vi "svx_Orbit Exec Commands.vi"(4 "Display State In":T2={"X Scale"={"Name"="Horizontal", "FString"="%#.2g", "Major Color"=16777238, "Minor Color"=16777216, "Scale Visible"=TRUE, " Label Visible"=TRUE, "Grid Style"=1}, "Y Scale"={"Name"="Vertical", "FString"="%#.2g", "Major Color"=16777238, "Minor Color"=16777216, "Scale Visible"=TRUE, " Label Visible"=TRUE, "Grid Style"=1}, "Plot"={"Point Style"=0, "Line Width"=0, "Line Style"=0, "Plot Color"=9727, "Point/fill"=0}, "Arrow/Crosshair Color"=9727, "Tacho Point Color"=16711680, "Container Bounds"={"Width"=563, "Height"=294}, "Axis Maximum"=10.0, "Probe Angles"={"Angle X"=0.0, "Angle Y"=1.5707963267948966}, "Background Color"=16777226, "Cursor"={"Cursor Point Style"=13, "Cursor Style"=4, "Cursor Line Width"=1, "Cursor Line Style"=0, "Cursor Color"=9727, "Cursor Name Visible"=TRUE, "Cursor Visible"=TRUE, "Cursor Position"={"X"=0.0, "Y"=0.0}, "Cursor Index"=0, "Cursor Lock"=FALSE}, "Elliptical Info"=[], "Legend Visible"=TRUE, "Scale Range Change"=refnum, "Strings[]"={"Custom pair name"=FALSE, "Row Strings []"=[], "Column Strings []"=[]}, "Index"=[{"pair index"=0, "order index"=0}], " Parents Tags"=[], "Children Tags"=[], "Open?"=[], "Label"="", "Legend Width"=120, "Pair Strings Changed?"=FALSE, "Size"=[], "Legend Background"=16777226, "Legend Font"=16777222, "Cursor Release"=refnum, "Autoscale"=TRUE, "Precession Direction"=[], "Item Width"=0, "User Pair Strings []"=[], "Users Order Strings []"=[], "Autoscale Once"=TRUE, "Property Write"=refnum} caption="State" {"Index"."order index" min=0; "Index"."pair index" min=0; "Axis Maximum" min=0.0}, 5 "Data In":T4, 6 "Commands":T1[](array[typedef]), 7 "Container":refnum<vi>, 8 "Facade VI":refnum<vi>, 9 "Cursor Info":refnum<vi>, 10 "Tree":refnum<vi>, 11 "Orbit Plot":refnum<vi>) -> (0 "Display State Out":T2={"X Scale"={"Name"="Horizontal", "FString"="%#.2g", "Major Color"=16777238, "Minor Color"=16777216, "Scale Visible"=TRUE, " Label Visible"=TRUE, "Grid Style"=1}, "Y Scale"={"Name"="Vertical", "FString"="%#.2g", "Major Color"=16777238, "Minor Color"=16777216, "Scale Visible"=TRUE, " Label Visible"=TRUE, "Grid Style"=1}, "Plot"={"Point Style"=0, "Line Width"=0, "Line Style"=0, "Plot Color"=9727, "Point/fill"=0}, "Arrow/Crosshair Color"=9727, "Tacho Point Color"=16711680, "Container Bounds"={"Width"=563, "Height"=294}, "Axis Maximum"=10.0, "Probe Angles"={"Angle X"=0.0, "Angle Y"=1.5707963267948966}, "Background Color"=16777226, "Cursor"={"Cursor Point Style"=13, "Cursor Style"=4, "Cursor Line Width"=1, "Cursor Line Style"=0, "Cursor Color"=9727, "Cursor Name Visible"=TRUE, "Cursor Visible"=TRUE, "Cursor Position"={"X"=0.0, "Y"=0.0}, "Cursor Index"=0, "Cursor Lock"=FALSE}, "Elliptical Info"=[], "Legend Visible"=TRUE, "Scale Range Change"=refnum, "Strings[]"={"Custom pair name"=FALSE, "Row Strings []"=[], "Column Strings []"=[]}, "Index"=[{"pair index"=0, "order index"=0}], " Parents Tags"=[], "Children Tags"=[], "Open?"=[], "Label"="", "Legend Width"=120, "Pair Strings Changed?"=FALSE, "Size"=[], "Legend Background"=16777226, "Legend Font"=16777222, "Cursor Release"=refnum, "Autoscale"=TRUE, "Precession Direction"=[], "Item Width"=0, "User Pair Strings []"=[], "Users Order Strings []"=[], "Autoscale Once"=TRUE, "Property Write"=refnum} caption="State" {"Index"."order index" min=0; "Index"."pair index" min=0; "Axis Maximum" min=0.0})   [LabVIEW 2017, in "SVX Orbit.xctl"]
uses:
  <vilib>/addons/_XControls/Orbit Plot/SVX Orbit.xctl
  <vilib>/addons/_XControls/Orbit Plot/subVIs/svx_Orbit Data.ctl
  <vilib>/addons/_XControls/Orbit Plot/subVIs/svx_Orbit Internal State.ctl
  <vilib>/addons/_XControls/Orbit Plot/subVIs/svx_Orbit Bounds.ctl
  <vilib>/addons/_XControls/Orbit Plot/subVIs/svx_Orbit Core States.ctl
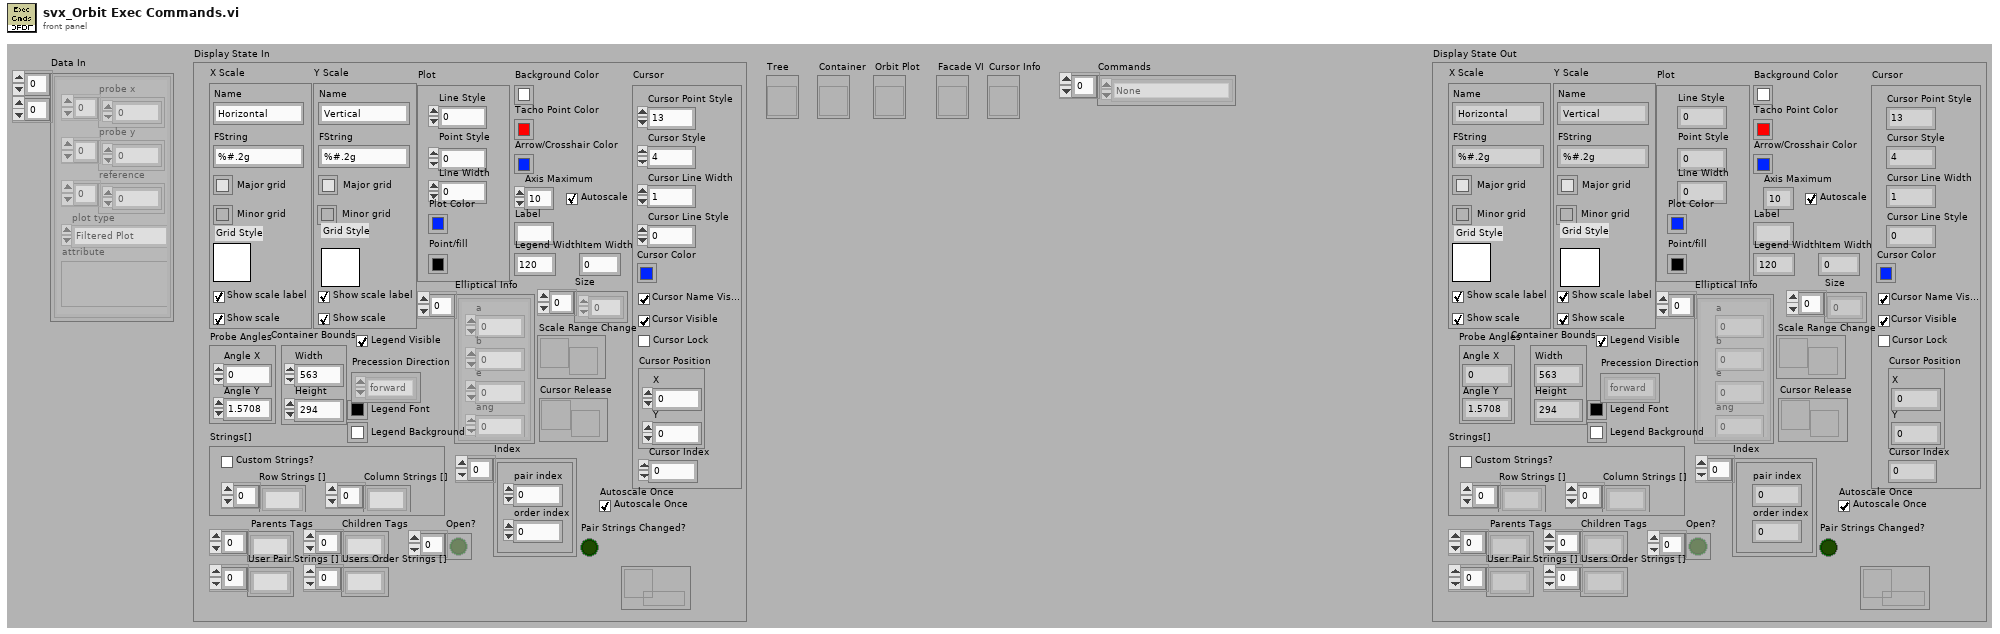
[diagram p1: front panel]
types:
  T1 = typedef "SVX Orbit.xctl/svx_Orbit Core States.ctl" = enum16{"None", "[Axis] Range", "[Plot] Image", "[Plot] Tacho Point", "[Plot] Grid and BG", "[Cursor] Cursor Info", "[Legend] Pair Strings", "[Data] Plot Data", "[Legend] Checkbox", "[Layout] Update", "[Legend] Tree Open", "[Layout] Legend Visible", "[Plot] Data Point", "[Axis] Axis and Label", "[Axis] Format String", "[Cursor] Appearance", "[Cursor] Index", "[Legend] Color", "[Layout] Min Pane Size", "[Data] Legend Strings"}
  T2 = typedef "SVX Orbit.xctl/svx_Orbit Internal State.ctl" = cluster{"X Scale":cluster{"Name":string, "FString":string, "Major Color":u32, "Minor Color":u32, "Scale Visible":bool, " Label Visible":bool, "Grid Style":u16}, "Y Scale":cluster{"Name":string, "FString":string, "Major Color":u32, "Minor Color":u32, "Scale Visible":bool, " Label Visible":bool, "Grid Style":u16}, "Plot":cluster{"Point Style":u8, "Line Width":u8, "Line Style":u8, "Plot Color":u32, "Point/fill":u32}, "Arrow/Crosshair Color":u32, "Tacho Point Color":u32, "Container Bounds":T3, "Axis Maximum":dbl, "Probe Angles":cluster{"Angle X":dbl, "Angle Y":dbl}, "Background Color":u32, "Cursor":cluster{"Cursor Point Style":u8, "Cursor Style":u8, "Cursor Line Width":u8, "Cursor Line Style":u8, "Cursor Color":u32, "Cursor Name Visible":bool, "Cursor Visible":bool, "Cursor Position":cluster{"X":dbl, "Y":dbl}, "Cursor Index":i32, "Cursor Lock":bool}, "Elliptical Info":cluster{"a":dbl, "b":dbl, "e":dbl, "ang":dbl}[], "Legend Visible":bool, "Scale Range Change":refnum<user-event>, "Strings[]":cluster{"Custom pair name":bool, "Row Strings []":string[], "Column Strings []":string[]}, "Index":cluster{"pair index":i32, "order index":i32}[], " Parents Tags":string[], "Children Tags":string[], "Open?":bool[], "Label":string, "Legend Width":u32, "Pair Strings Changed?":bool, "Size":i32[], "Legend Background":u32, "Legend Font":u32, "Cursor Release":refnum<user-event>, "Autoscale":bool, "Precession Direction":enum16{"forward", "backward"}[], "Item Width":u32, "User Pair Strings []":string[], "Users Order Strings []":string[], "Autoscale Once":bool, "Property Write":refnum<queue>}
  T3 = typedef "SVX Orbit.xctl/svx_Orbit Bounds.ctl" = cluster{"Width":u32, "Height":u32}
  T4 = typedef "SVX Orbit.xctl/svx_Orbit Data.ctl" = cluster{"probe x":dbl[], "probe y":dbl[], "reference":dbl[], "plot type":enum16{"Filtered Plot", "Unfiltered Plot"}, "attribute":variant}[][]
  T5 = cluster{"probe x":dbl[], "probe y":dbl[], "reference":dbl[], "plot type":enum16{"Filtered Plot", "Unfiltered Plot"}, "attribute":variant}
  T6 = typedef "LVBoundsTypeDef.ctl" = cluster{"Width":u32, "Height":u32}
  T7 = cluster{"Cursor Point Style":u8, "Cursor Style":u8, "Cursor Line Width":u8, "Cursor Line Style":u8, "Cursor Color":u32, "Cursor Name Visible":bool, "Cursor Visible":bool, "Cursor Position":cluster{"X":dbl, "Y":dbl}, "Cursor Index":i32, "Cursor Lock":bool}
  T8 = typedef "LVPointDoubleTypeDef.ctl" = cluster{"Cursor X":dbl, "Cursor Y":dbl}
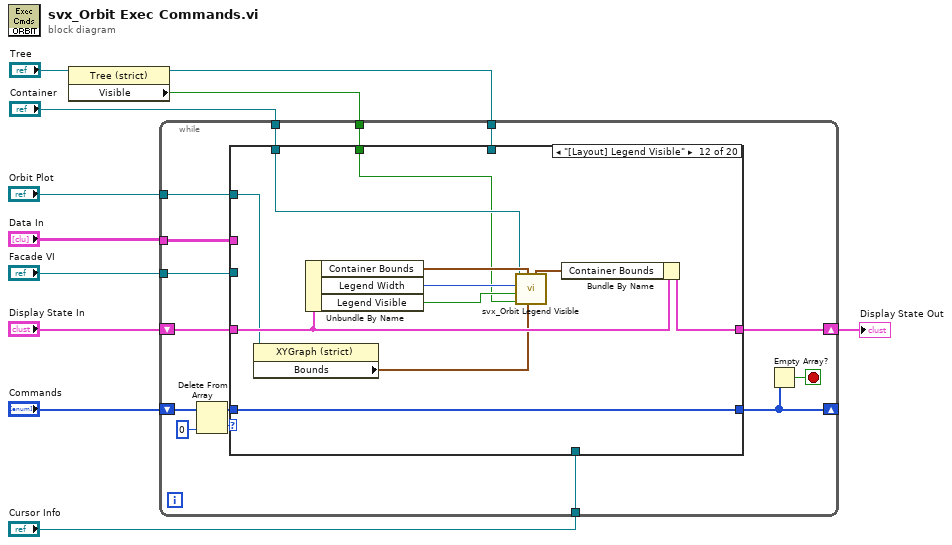
[diagram p0: block diagram]
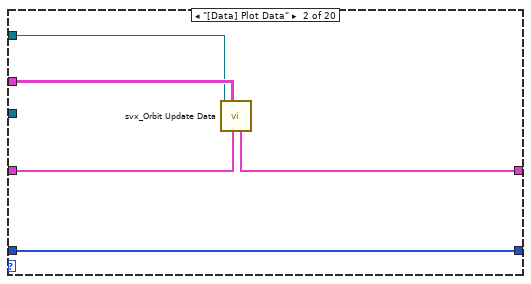
[diagram p3: hidden frame]
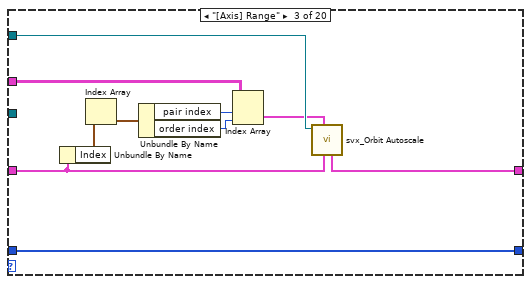
[diagram p4: hidden frame]
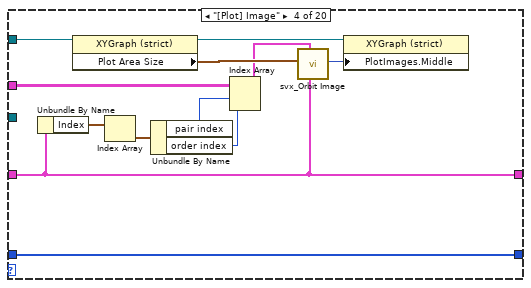
[diagram p5: hidden frame]
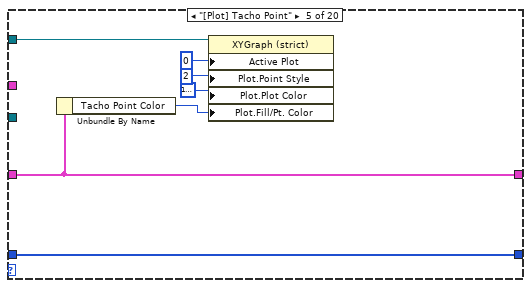
[diagram p6: hidden frame]
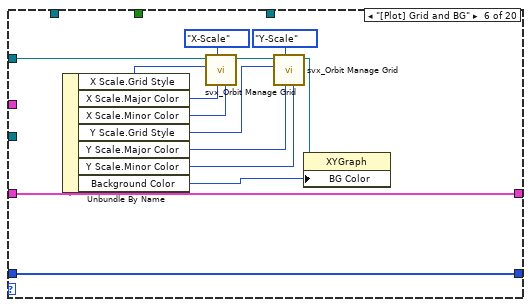
[diagram p7: hidden frame]
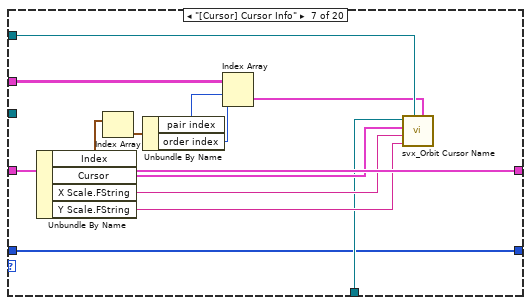
[diagram p8: hidden frame]
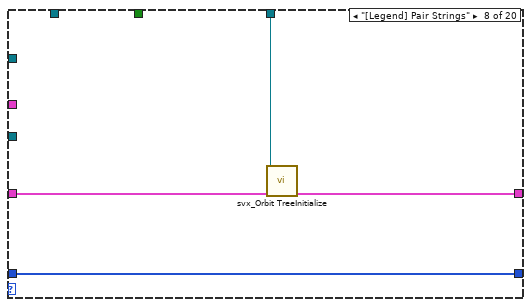
[diagram p9: hidden frame]
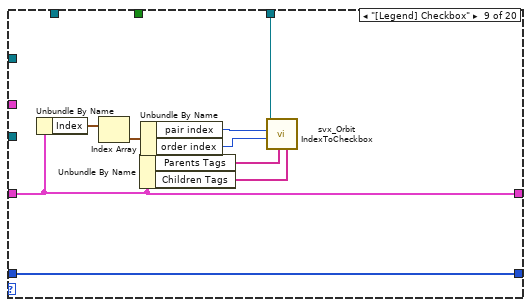
[diagram p10: hidden frame]
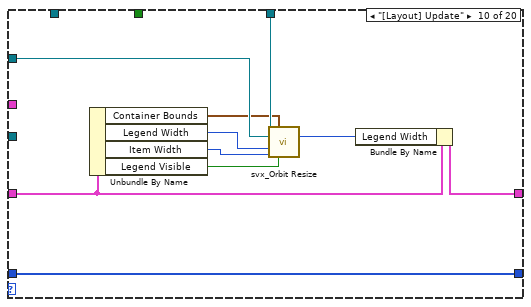
[diagram p11: hidden frame]
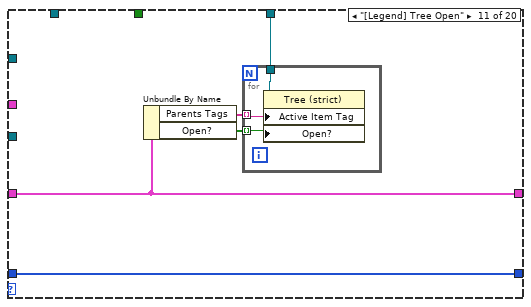
[diagram p12: hidden frame]
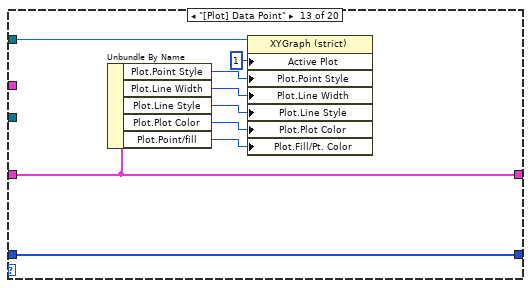
[diagram p13: hidden frame]
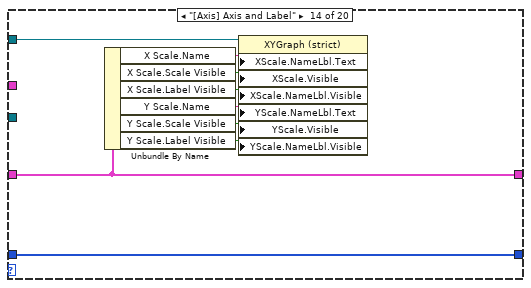
[diagram p14: hidden frame]
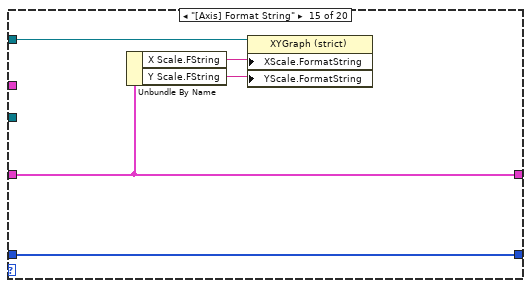
[diagram p15: hidden frame]
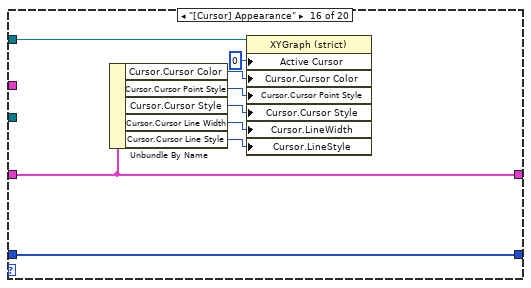
[diagram p16: hidden frame]
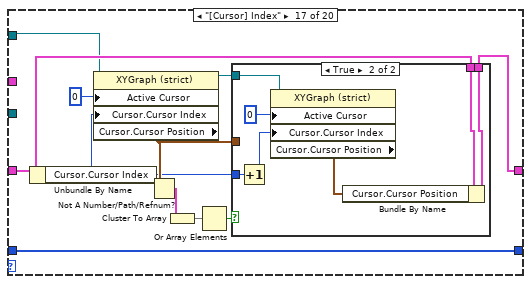
[diagram p17: hidden frame]
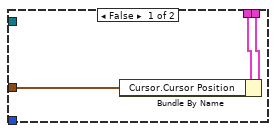
[diagram p18: hidden frame]
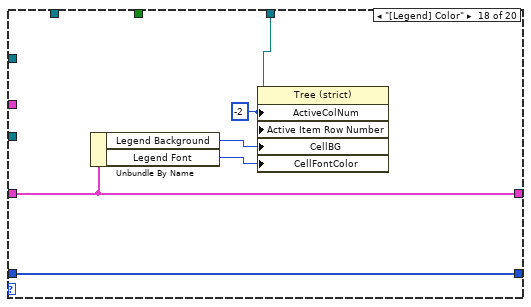
[diagram p19: hidden frame]
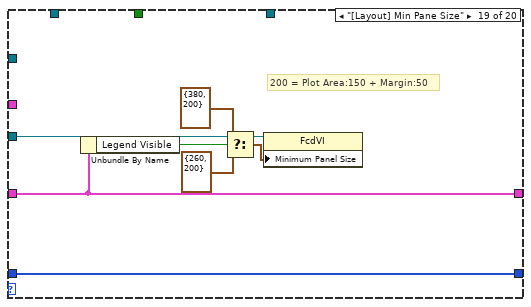
[diagram p20: hidden frame]
diagram:
  n1 = property class="Tree (strict)"(reference="Tree") -> (reference out=w3:refnum<vi>, "Visible"=w1:bool)  [unwired: 1 in, 1 out]
  n2 = while {
    shift-right: [w24] -> w7
    shift-left: "Display State In" -> [w25]
    tunnel: "Data In" -> [w23]
    tunnel: "Orbit Plot" -> [w22]
    tunnel: "Container" -> [w21]
    tunnel: w3 -> [w20]
    tunnel: "Facade VI" -> [w19]
    tunnel: "Cursor Info" -> [w18]
    shift-right: [w15] -> _
    shift-left: "Commands" -> [w26]
    tunnel: w1 -> [w12]
    stop <- w14 stop-if-true
    n3 = Delete From Array(array=w26, index=0 ("length")) -> (deleted portion=w17:T1, array with subset deleted=w16:T1[])  [unwired: 1 in]
    n4 = case shown="\"[Layout] Legend Visible\"" w17 {
      tunnel: w25 -> [w28 w33 w35 w48 w62 w66 w88 w93 w94 w106 w117 w129 w140 w146 w151 w157 w167 w187 w194 w207]
      tunnel: [w28 w32 w34 w48 w62 w66 w88 w92 w94 w104 w117 w128 w140 w146 w151 w157 w168 w187 w194 w206] -> w24
      tunnel: w23 -> [_ w30 w40 w46 _ _ w77 _ _ _ _ _ _ _ _ _ _ _ _ w208]
      tunnel: w22 -> [_ w29 w43 w53 w57 w67 w89 _ _ w112 _ w122 w139 w145 w153 w163 w165 _ _ _]
      tunnel: w21 -> [_ _ _ _ _ _ _ _ _ _ _ w130 _ _ _ _ _ _ _ _]
      tunnel: w20 -> [_ _ _ _ _ _ _ w91 w100 w108 w114 _ _ _ _ _ _ w186 _ _]
      tunnel: w19 -> [_ _ _ _ _ _ _ _ _ _ _ _ _ _ _ _ _ _ w195 _]
      tunnel: w18 -> [_ _ _ _ _ _ w84 _ _ _ _ _ _ _ _ _ _ _ _ _]
      tunnel: w16 -> [w27 w31 w42 w51 w56 w63 w83 w90 w99 w107 w115 w126 w132 w141 w150 w156 w166 w185 w191 w201]
      tunnel: [w27 w31 w42 w51 w56 w63 w83 w90 w99 w107 w115 w126 w132 w141 w150 w156 w166 w185 w191 w205] -> w15
      tunnel: w12 -> [_ _ _ _ _ _ _ _ _ _ _ w124 _ _ _ _ _ _ _ _]
      frame "None", Default {
      }
      frame "[Data] Plot Data" {
        n5 = call <vilib>:"svx_Orbit Update Data.vi"("State in"=w33, "orbit plot"=w30, "Orbit Plot"=w29) -> ("State out"=w32:T2)  [unwired: 8 in]
      }
      frame "[Axis] Range" {
        n6 = Unbundle By Name(w35) -> ("Index"=w41:cluster{"pair index":i32, "order index":i32}[])
        n7 = Index Array(array=w41) -> (element=w39:cluster{"pair index":i32, "order index":i32})  [unwired: 1 in]
        n8 = Unbundle By Name(w39) -> ("pair index"=w38:i32, "order index"=w37:i32)
        n9 = Index Array(array=w40, index (row)=w38, index (col)=w37) -> (element=w36:T5)
        n10 = call <vilib>:"svx_Orbit Autoscale.vi"("Display State In"=w35, 7:"Orbit Plot"=w36, 11:"Orbit Plot"=w43) -> ("Display State Out"=w34:T2)  [unwired: 8 in]
      }
      frame "[Plot] Image" {
        n11 = Unbundle By Name(w48) -> ("Index"=w47:cluster{"pair index":i32, "order index":i32}[])
        n12 = property on="Property Node" class="XYGraph (strict)"(reference=w53) -> (reference out=w52:refnum<vi>, "Plot Area Size"=w54:T6)  [unwired: 1 in, 1 out]
        n13 = Index Array(array=w47) -> (element=w50:cluster{"pair index":i32, "order index":i32})  [unwired: 1 in]
        n14 = Unbundle By Name(w50) -> ("pair index"=w49:i32, "order index"=w45:i32)
        n15 = Index Array(array=w46, index (row)=w49, index (col)=w45) -> (element=w44:T5)
        n16 = call <vilib>:"svx_Orbit Image.vi"("State"=w48, "Orbit Plot"=w44, "Plot Area:Size"=w54) -> ("Picture Out"=w55:picture)  [unwired: 8 in]
        n17 = property on="Property Node" class="XYGraph (strict)"(reference=w52, "PlotImages.Middle"=w55) -> ()  [unwired: 1 in, 2 out]
      }
      frame "[Plot] Tacho Point" {
        n18 = Unbundle By Name(w62) -> ("Tacho Point Color"=w60:u32)
        n19 = property on="Property Node" class="XYGraph (strict)"(reference=w57, "Active Plot"=u32 0, "Plot.Point Style"=u8 2, "Plot.Plot Color"=u32 16777216, "Plot.Fill/Pt. Color"=w60) -> ()  [unwired: 1 in, 2 out]
      }
      frame "[Plot] Grid and BG" {
        n20 = Unbundle By Name(w66) -> ("X Scale.Grid Style"=w76:u16, "X Scale.Major Color"=w75:u32, "X Scale.Minor Color"=w74:u32, "Y Scale.Grid Style"=w73:u16, "Y Scale.Major Color"=w71:u32, "Y Scale.Minor Color"=w70:u32, "Background Color"=w64:u32)
        n21 = call <vilib>:"svx_Orbit Manage Grid.vi"("Minor Color"=w74, "Major Color"=w75, "Axis"=enum16{"X-Scale", "Y-Scale", "Z-Scale"}."X-Scale", "Grid Style"=w76, "Orbit Plot"=w67) -> ("Orbit Plot out"=w72:refnum<vi>)  [unwired: 4 in, 2 out]
        n22 = call <vilib>:"svx_Orbit Manage Grid.vi"("Minor Color"=w70, "Major Color"=w71, "Axis"=enum16{"X-Scale", "Y-Scale", "Z-Scale"}."Y-Scale", "Grid Style"=w73, "Orbit Plot"=w72) -> ("Orbit Plot out"=w65:refnum<vi>)  [unwired: 4 in, 2 out]
        n23 = property class="XYGraph"(reference=w65, "BG Color"=w64) -> ()  [unwired: 1 in, 2 out]
      }
      frame "[Cursor] Cursor Info" {
        n24 = Unbundle By Name(w88) -> ("Index"=w80:cluster{"pair index":i32, "order index":i32}[], "Cursor"=w87:T7, "X Scale.FString"=w86:string, "Y Scale.FString"=w85:string)
        n25 = Index Array(array=w80) -> (element=w82:cluster{"pair index":i32, "order index":i32})  [unwired: 1 in]
        n26 = Unbundle By Name(w82) -> ("pair index"=w81:i32, "order index"=w79:i32)
        n27 = Index Array(array=w77, index (row)=w81, index (col)=w79) -> (element=w78:T5)
        n28 = call <vilib>:"svx_Orbit Cursor Name.vi"(5:"Orbit Plot"=w78, 7:"Orbit Plot"=w89, "Y FString"=w85, "X FString"=w86, "Cursor"=w87, "Cursor Info"=w84) -> ()  [unwired: 6 in]
      }
      frame "[Legend] Pair Strings" {
        n29 = call <vilib>:"svx_Orbit TreeInitialize.vi"("State in"=w93, "Tree ref in"=w91) -> ("State out"=w92:T2)  [unwired: 8 in, 1 out]
      }
      frame "[Legend] Checkbox" {
        n30 = Unbundle By Name(w94) -> ("Index"=w97:cluster{"pair index":i32, "order index":i32}[])
        n31 = Index Array(array=w97) -> (element=w98:cluster{"pair index":i32, "order index":i32})  [unwired: 1 in]
        n32 = Unbundle By Name(w94) -> ("Parents Tags"=w102:string[], "Children Tags"=w101:string[])
        n33 = Unbundle By Name(w98) -> ("pair index"=w96:i32, "order index"=w95:i32)
        n34 = call <vilib>:"svx_Orbit IndexToCheckbox.vi"("All Children Tags"=w101, "All parents Tags"=w102, "ColumnIdx"=w95, "RowIdx"=w96, "Tree ref in"=w100) -> ()  [unwired: 6 in, 1 out]
      }
      frame "[Layout] Update" {
        n35 = Unbundle By Name(w106) -> ("Container Bounds"=w105:T3, "Legend Width"=w110:u32, "Item Width"=w109:u32, "Legend Visible"=w111:bool)
        n36 = call <vilib>:"svx_Orbit Resize.vi"("Container Bounds"=w105, "XY"=w112, "Tree ref in"=w108, "Legend Width"=w110, "Item Width"=w109, "Legend Visible"=w111) -> ("Width"=w103:u32)  [unwired: 9 in]
        n37 = Bundle By Name(cluster=w106, "Legend Width"=w103) -> (w104:T2)
      }
      frame "[Legend] Tree Open" {
        n38 = Unbundle By Name(w117) -> ("Parents Tags"=w113:string[], "Open?"=w116:bool[])
        n39 = for {
          tunnel: w113 -> [w120] mode=indexing
          tunnel: w116 -> [w119] mode=indexing
          tunnel: w114 -> [w118]
          n40 = property on="Property Node" class="Tree (strict)"(reference=w118, "Active Item Tag"=w120, "Open?"=w119) -> ()  [unwired: 1 in, 2 out]
        }
      }
      frame "[Layout] Legend Visible" {
        n41 = property class="XYGraph (strict)"(reference=w122) -> ("Bounds"=w121:T6)  [unwired: 1 in, 2 out]
        n42 = Unbundle By Name(w129) -> ("Container Bounds"=w131:T3, "Legend Width"=w127:u32, "Legend Visible"=w125:bool)
        n43 = call <vilib>:"svx_Orbit Legend Visible.vi"("Bounds"=w121, "Bounds In"=w131, "Previous Visible?"=w124, "Legend Visible"=w125, "Legend Width"=w127, "Container"=w130) -> ("Bounds Out"=w123:cluster{"Width":u32, u32})  [unwired: 5 in]
        n44 = Bundle By Name(cluster=w129, "Container Bounds"=w123) -> (w128:T2)
      }
      frame "[Plot] Data Point" {
        n45 = Unbundle By Name(w140) -> ("Plot.Point Style"=w134:u8, "Plot.Line Width"=w135:u8, "Plot.Line Style"=w136:u8, "Plot.Plot Color"=w137:u32, "Plot.Point/fill"=w138:u32)
        n46 = property on="Property Node" class="XYGraph (strict)"(reference=w139, "Active Plot"=u32 1, "Plot.Point Style"=w134, "Plot.Line Width"=w135, "Plot.Line Style"=w136, "Plot.Plot Color"=w137, "Plot.Fill/Pt. Color"=w138) -> ()  [unwired: 1 in, 2 out]
      }
      frame "[Axis] Axis and Label" {
        n47 = Unbundle By Name(w146) -> ("X Scale.Name"=w144:string, "X Scale.Scale Visible"=w147:bool, "X Scale.Label Visible"=w148:bool, "Y Scale.Name"=w142:string, "Y Scale.Scale Visible"=w143:bool, "Y Scale.Label Visible"=w149:bool)
        n48 = property on="Property Node" class="XYGraph (strict)"(reference=w145, "XScale.NameLbl.Text"=w144, "XScale.Visible"=w147, "XScale.NameLbl.Visible"=w148, "YScale.NameLbl.Text"=w142, "YScale.Visible"=w143, "YScale.NameLbl.Visible"=w149) -> ()  [unwired: 1 in, 2 out]
      }
      frame "[Axis] Format String" {
        n49 = Unbundle By Name(w151) -> ("X Scale.FString"=w154:string, "Y Scale.FString"=w152:string)
        n50 = property on="Property Node" class="XYGraph (strict)"(reference=w153, "XScale.FormatString"=w154, "YScale.FormatString"=w152) -> ()  [unwired: 1 in, 2 out]
      }
      frame "[Cursor] Appearance" {
        n51 = Unbundle By Name(w157) -> ("Cursor.Cursor Color"=w162:u32, "Cursor.Cursor Point Style"=w161:u8, "Cursor.Cursor Style"=w160:u8, "Cursor.Cursor Line Width"=w159:u8, "Cursor.Cursor Line Style"=w158:u8)
        n52 = property on="Property Node" class="XYGraph (strict)"(reference=w163, "Active Cursor"=u32 0, "Cursor.Cursor Color"=w162, "Cursor.Cursor Point Style"=w161, "Cursor.Cursor Style"=w160, "Cursor.LineWidth"=w159, "Cursor.LineStyle"=w158) -> ()  [unwired: 1 in, 2 out]
      }
      frame "[Cursor] Index" {
        n53 = Unbundle By Name(w167) -> ("Cursor.Cursor Index"=w170:i32)
        n54 = property on="Property Node" class="XYGraph (strict)"(reference=w165, "Active Cursor"=u32 0, "Cursor.Cursor Index"=w170) -> (reference out=w164:refnum<vi>, "Cursor.Cursor Position"=w171:T8)  [unwired: 1 in, 1 out]
        n55 = Not A Number/Path/Refnum?(number/path/refnum=w171) -> (NaN/Path/Refnum?=w172:cluster{"Cursor X":bool, "Cursor Y":bool})
        n56 = Cluster To Array(cluster=w172) -> (array=w173:bool[])
        n57 = Or Array Elements(Boolean array=w173) -> (logical OR=w174:bool)
        n58 = case shown="True" w174 {
          tunnel: w167 -> [w177 w184]
          tunnel: [w176 w183] -> w168
          tunnel: w170 -> [_ w181]
          tunnel: w171 -> [w175 _]
          tunnel: w164 -> [_ w178]
          frame False {
            n59 = Bundle By Name(cluster=w177, "Cursor.Cursor Position"=w175) -> (w176:T2)
          }
          frame True {
            n60 = Increment(x=w181) -> (x+1=w180:i32)
            n61 = property on="Property Node" class="XYGraph (strict)"(reference=w178, "Active Cursor"=u32 0, "Cursor.Cursor Index"=w180) -> ("Cursor.Cursor Position"=w179:T8)  [unwired: 1 in, 2 out]
            n62 = Bundle By Name(cluster=w184, "Cursor.Cursor Position"=w179) -> (w183:T2)
          }
        }
      }
      frame "[Legend] Color" {
        w188 = -2 ("Active Cell:Active Column Number")
        n63 = Unbundle By Name(w187) -> ("Legend Background"=w189:u32, "Legend Font"=w190:u32)
        n64 = property on="Property Node" class="Tree (strict)"(reference=w186, "ActiveColNum"=w188, "Active Item Row Number"=w188, "CellBG"=w189, "CellFontColor"=w190) -> ()  [unwired: 1 in, 2 out]
      }
      frame "[Layout] Min Pane Size" {
        # "200 = Plot Area:150 + Margin:50"
        n65 = Unbundle By Name(w194) -> ("Legend Visible"=w193:bool)
        n66 = Select(t=cluster{"Horizontal":i16, "Vertical":i16} {"Horizontal"=380, "Vertical"=200} ("Front Panel Window:Minimum Size"), s=w193, f=cluster{"Horizontal":i16, "Vertical":i16} {"Horizontal"=260, "Vertical"=200}) -> (s? t:f=w197:cluster{"Horizontal":i16, "Vertical":i16})
        n67 = property class="FcdVI"(reference=w195, "Minimum Panel Size"=w197) -> ()  [unwired: 1 in, 2 out]
      }
      frame "[Data] Legend Strings" {
        w202 = T1[] [] items=["None", "[Axis] Range", "[Plot] Image", "[Plot] Tacho Point", "[Plot] Grid and BG", "[Cursor] Cursor Info", "[Legend] Pair Strings", "[Data] Plot Data", "[Legend] Checkbox", "[Layout] Update", "[Legend] Tree Open", "[Layout] Legend Visible", "[Plot] Data Point", "[Axis] Axis and Label", "[Axis] Format String", "[Cursor] Appearance", "[Cursor] Index", "[Legend] Color", "[Layout] Min Pane Size", "[Data] Legend Strings"]
        w203 = T1[] [enum."[Legend] Pair Strings", enum."[Legend] Checkbox", enum."[Legend] Tree Open"] items=["None", "[Axis] Range", "[Plot] Image", "[Plot] Tacho Point", "[Plot] Grid and BG", "[Cursor] Cursor Info", "[Legend] Pair Strings", "[Data] Plot Data", "[Legend] Checkbox", "[Layout] Update", "[Legend] Tree Open", "[Layout] Legend Visible", "[Plot] Data Point", "[Axis] Axis and Label", "[Axis] Format String", "[Cursor] Appearance", "[Cursor] Index", "[Legend] Color", "[Layout] Min Pane Size", "[Data] Legend Strings"]
        n68 = call <vilib>:"svx_Orbit Update Pair.vi"("State in"=w207, "Label.Text"="Orbit Plot", "orbit plot"=w208) -> ("update tree?"=w204:bool, "State out"=w206:T2)  [unwired: 7 in]
        n69 = Select(t=w203, s=w204, f=w202) -> (s? t:f=w199:T1[])
        n70 = for {
          shift-right: [w210] -> w200
          shift-left: w201 -> [w211]
          tunnel: w199 -> [w209] mode=indexing
          n71 = Search 1D Array(1D array=w211, element=w209) -> (index of element=w213:i32)  [unwired: 1 in]
          n72 = Delete From Array(array=w211, length=1, index=w213) -> (array with subset deleted=w210:T1[])  [unwired: 1 out]
        }
        n73 = Build Array (concatenate)(w200, w199) -> (w205:T1[])
      }
    }
    n74 = Empty Array?(array=w15) -> (empty?=w14:bool)
  }
  "Display State Out" <- w7
